vi "[GV]_E-STOP.vi"() -> ()   [LabVIEW 2016]
panel:
  in  "E-STOP":bool
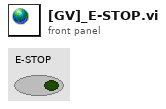
[diagram p1: front panel]
diagram:
